vi "SettingsToRegisters.vi"(4 "LP_LowerLimit":u32=644245094 format="%x", 5 "LP_UpperLimit":u32=1073741824 format="%x", 6 "HP_LowerLimit":u32=590558003 format="%x", 7 "HP_UpperLimit":u32=1020054732 format="%x", 10 "WriteSize":enum16{"1", "2", "4"}(ring)=enum."4", 11 "coordinates":T1 {"YLP_RR" format="%x"; "YLP_FR" format="%x"; "YHP_RR" format="%x"; "YHP_FR" format="%x"; "XLP_RR" format="%x"; "XLP_FR" format="%x"; "XHPstart" format="%x"; "XHPend" format="%x"; "XLPstart" format="%x"; "XLPend" format="%x"; "YHPstart" format="%x"; "YHPend" format="%x"; "YLPstart" format="%x"; "YLPend" format="%x"; "XHP_RR" format="%x"; "XHP_FR" format="%x"}) -> (1 "OutOfRange":bool, 2 "size(s)":i32, 3 "Register Writes":cluster{"Address":u8, "Value":u32}[](array[cluster]))   [LabVIEW 2014]
uses:
  CoordinateSettings.ctl
panel:
  out "WriteLength":i16=15
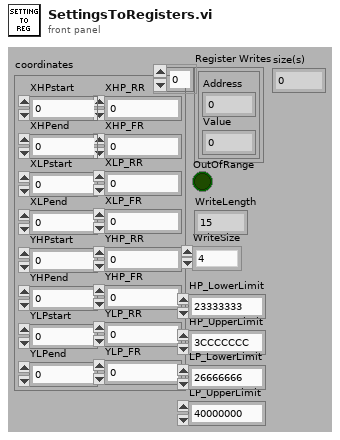
[diagram p1: front panel]
types:
  T1 = typedef "CoordinateSettings.ctl" = cluster{"XHPstart":u32, "XHPend":u32, "XLPstart":u32, "XLPend":u32, "YHPstart":u32, "YHPend":u32, "YLPstart":u32, "YLPend":u32, "XHP_RR":u32, "XHP_FR":u32, "XLP_FR":u32, "XLP_RR":u32, "YHP_FR":u32, "YHP_RR":u32, "YLP_FR":u32, "YLP_RR":u32}
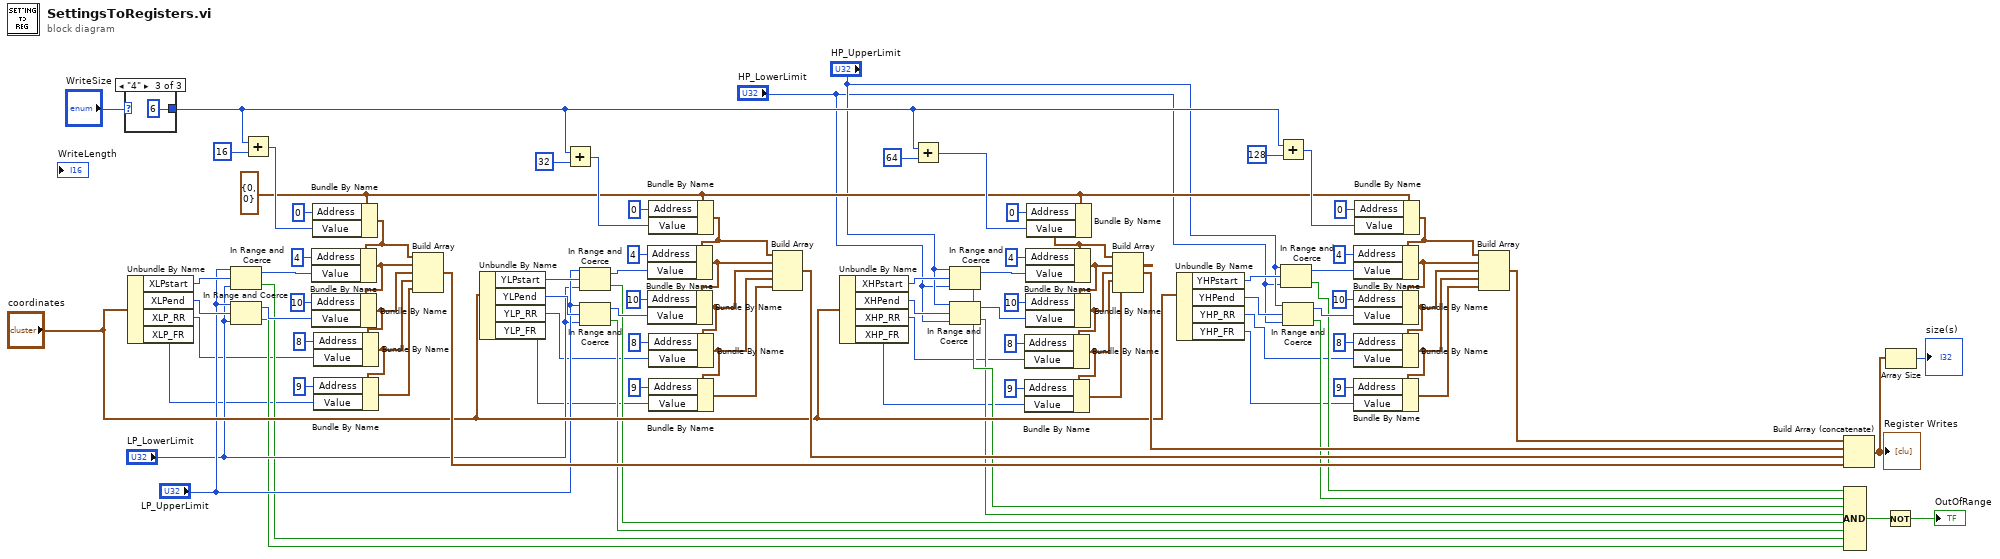
[diagram p0: block diagram]
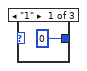
[diagram p2: hidden frame]
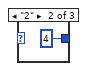
[diagram p3: hidden frame]
diagram:
  w63 = cluster{"Address":u8, "Value":u32} {"Address"=0, "Value"=0}
  n1 = case shown="\"4\"" "WriteSize" {
    tunnel: [u8 0 u8 4 u8 6] -> w62
    frame "1" {
    }
    frame "2" {
    }
    frame "4" {
    }
  }
  n2 = Unbundle By Name("coordinates") -> ("XLPstart"=w50:u32, "XLPend"=w49:u32, "XLP_RR"=w27:u32, "XLP_FR"=w26:u32)
  n3 = In Range and Coerce(upper limit="LP_UpperLimit", x=w50, lower limit="LP_LowerLimit") -> (coerced(x)=w48:u32, In Range?=w34:bool)
  n4 = In Range and Coerce(upper limit="LP_UpperLimit", x=w49, lower limit="LP_LowerLimit") -> (coerced(x)=w47:u32, In Range?=w33:bool)
  n5 = Add(x=w62, y=u8 16) -> (x+y=w70:u8)
  n6 = Bundle By Name(cluster=w63, "Address"=u8 0, "Value"=w70) -> (w93:cluster{"Address":u8, "Value":u32})
  n7 = Bundle By Name(cluster=w93, "Address"=u8 4, "Value"=w48) -> (w92:cluster{"Address":u8, "Value":u32})
  n8 = Bundle By Name(cluster=w92, "Address"=u8 10, "Value"=w47) -> (w28:cluster{"Address":u8, "Value":u32})
  n9 = Bundle By Name(cluster=w28, "Address"=u8 8, "Value"=w27) -> (w25:cluster{"Address":u8, "Value":u32})
  n10 = Bundle By Name(cluster=w25, "Address"=u8 9, "Value"=w26) -> (w24:cluster{"Address":u8, "Value":u32})
  n11 = Build Array(w93, w92, w28, w25, w24) -> (w73:cluster{"Address":u8, "Value":u32}[])
  n12 = Unbundle By Name("coordinates") -> ("YLPstart"=w46:u32, "YLPend"=w45:u32, "YLP_RR"=w18:u32, "YLP_FR"=w17:u32)
  n13 = Add(x=w62, y=u8 32) -> (x+y=w68:u8)
  n14 = In Range and Coerce(upper limit="LP_UpperLimit", x=w46, lower limit="LP_LowerLimit") -> (coerced(x)=w44:u32, In Range?=w36:bool)
  n15 = In Range and Coerce(upper limit="LP_UpperLimit", x=w45, lower limit="LP_LowerLimit") -> (coerced(x)=w43:u32, In Range?=w35:bool)
  n16 = Bundle By Name(cluster=w63, "Address"=u8 0, "Value"=w68) -> (w88:cluster{"Address":u8, "Value":u32})
  n17 = Bundle By Name(cluster=w88, "Address"=u8 4, "Value"=w44) -> (w87:cluster{"Address":u8, "Value":u32})
  n18 = Bundle By Name(cluster=w87, "Address"=u8 10, "Value"=w43) -> (w21:cluster{"Address":u8, "Value":u32})
  n19 = Bundle By Name(cluster=w21, "Address"=u8 8, "Value"=w18) -> (w20:cluster{"Address":u8, "Value":u32})
  n20 = Bundle By Name(cluster=w20, "Address"=u8 9, "Value"=w17) -> (w19:cluster{"Address":u8, "Value":u32})
  n21 = Build Array(w88, w87, w21, w20, w19) -> (w74:cluster{"Address":u8, "Value":u32}[])
  n22 = Unbundle By Name("coordinates") -> ("XHPstart"=w60:u32, "XHPend"=w57:u32, "XHP_RR"=w11:u32, "XHP_FR"=w10:u32)
  n23 = Add(x=w62, y=u8 64) -> (x+y=w66:u8)
  n24 = In Range and Coerce(upper limit="HP_UpperLimit", x=w60, lower limit="HP_LowerLimit") -> (coerced(x)=w59:u32, In Range?=w38:bool)
  n25 = In Range and Coerce(upper limit="HP_UpperLimit", x=w57, lower limit="HP_LowerLimit") -> (coerced(x)=w58:u32, In Range?=w37:bool)
  n26 = Bundle By Name(cluster=w63, "Address"=u8 0, "Value"=w66) -> (w83:cluster{"Address":u8, "Value":u32})
  n27 = Bundle By Name(cluster=w83, "Address"=u8 4, "Value"=w59) -> (w82:cluster{"Address":u8, "Value":u32})
  n28 = Bundle By Name(cluster=w82, "Address"=u8 10, "Value"=w58) -> (w14:cluster{"Address":u8, "Value":u32})
  n29 = Bundle By Name(cluster=w14, "Address"=u8 8, "Value"=w11) -> (w13:cluster{"Address":u8, "Value":u32})
  n30 = Bundle By Name(cluster=w13, "Address"=u8 9, "Value"=w10) -> (w12:cluster{"Address":u8, "Value":u32})
  n31 = Build Array(w83, w82, w14, w13, w12) -> (w75:cluster{"Address":u8, "Value":u32}[])
  n32 = Unbundle By Name("coordinates") -> ("YHPstart"=w56:u32, "YHPend"=w55:u32, "YHP_RR"=w4:u32, "YHP_FR"=w3:u32)
  n33 = Add(x=w62, y=u8 128) -> (x+y=w64:u8)
  n34 = In Range and Coerce(upper limit="HP_UpperLimit", x=w56, lower limit="HP_LowerLimit") -> (coerced(x)=w53:u32, In Range?=w40:bool)
  n35 = In Range and Coerce(upper limit="HP_UpperLimit", x=w55, lower limit="HP_LowerLimit") -> (coerced(x)=w54:u32, In Range?=w39:bool)
  n36 = Bundle By Name(cluster=w63, "Address"=u8 0, "Value"=w64) -> (w78:cluster{"Address":u8, "Value":u32})
  n37 = Bundle By Name(cluster=w78, "Address"=u8 4, "Value"=w53) -> (w77:cluster{"Address":u8, "Value":u32})
  n38 = Bundle By Name(cluster=w77, "Address"=u8 10, "Value"=w54) -> (w7:cluster{"Address":u8, "Value":u32})
  n39 = Bundle By Name(cluster=w7, "Address"=u8 8, "Value"=w4) -> (w6:cluster{"Address":u8, "Value":u32})
  n40 = Bundle By Name(cluster=w6, "Address"=u8 9, "Value"=w3) -> (w5:cluster{"Address":u8, "Value":u32})
  n41 = Build Array(w78, w77, w7, w6, w5) -> (w76:cluster{"Address":u8, "Value":u32}[])
  n42 = Build Array (concatenate)(w76, w75, w74, w73) -> (w2:cluster{"Address":u8, "Value":u32}[])
  "Register Writes" <- w2
  n43 = Compound Arithmetic op=AND(w40, w39, w38, w37, w36, w35, w34, w33) -> (w32:bool)
  n44 = Not(x=w32) -> (.not. x?=→"OutOfRange":bool)
  n45 = Array Size(array=w2) -> (size(s)=→"size(s)":i32)
